vi "GetWireTerminals.vi"(5 "Wire in":refnum<class "Wire.lvclass">, 6 "error in":errorcluster, 9 "VI Interpreter in":refnum<class "VI Interpreter.lvclass">) -> (0 "error out":errorcluster, 3 "VI Interpreter out":refnum<class "VI Interpreter.lvclass">, 4 "Wire out":refnum<class "Wire.lvclass">)   [LabVIEW 2014, in "VI Interpreter.lvclass"]
uses:
  VI Interpreter.lvclass
  Wire/Wire.lvclass
  Terminal/Terminal.lvclass
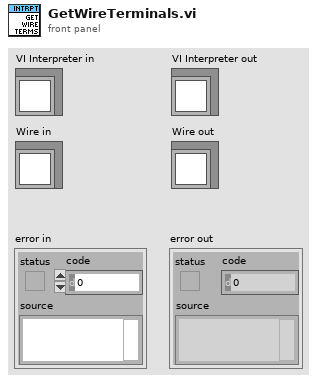
[diagram p1: front panel]
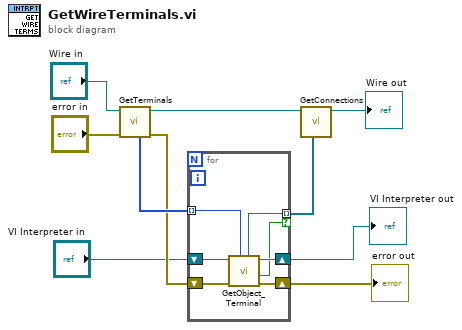
[diagram p0: block diagram]
diagram:
  n1 = call "GetTerminals.vi"("error in"="error in", "Wire in"="Wire in") -> ("error out"=w9:errorcluster, "Wire out"=w3:refnum<class "Wire.lvclass">, "terminals"=w10:i32[])  [unwired: 5 in]
  n2 = for {
    shift-right: [w13] -> w8
    shift-left: "VI Interpreter in" -> [w17]
    tunnel: w10 -> [w16] mode=indexing
    shift-right: [w15] -> w7
    shift-left: w9 -> [w14]
    tunnel: [w12] -> w1 mode=indexing if=w11
    n3 = call "GetObject_Terminal.vi"("UID"=w16, "error in"=w14, "VI Interpreter in"=w17) -> ("error out"=w15:errorcluster, "found"=w11:bool, "VI Interpreter out"=w13:refnum<class "VI Interpreter.lvclass">, "Terminal"=w12:refnum<class "Terminal.lvclass">)  [unwired: 3 in]
  }
  "error out" <- w7
  "VI Interpreter out" <- w8
  n4 = call "GetConnections.vi"("Terminals"=w1, "Wire in"=w3) -> ("Wire out"=→"Wire out":refnum<class "Wire.lvclass">)  [unwired: 7 in]
